vi "Check Condition.vi"(1 "Dictance":dbl, 2 "Condition":dbl, 3 "Reset":bool) -> (0 "Done":bool)   [LabVIEW 2015]
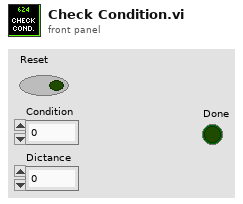
[diagram p1: front panel]
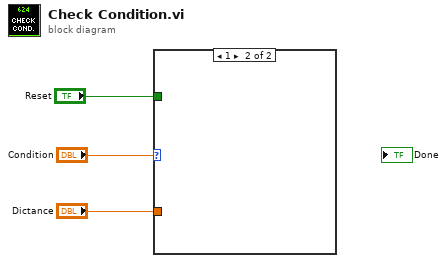
[diagram p0: block diagram]
diagram:
  n1 = case shown="1" "Condition" {
    tunnel: "Dictance" -> [_ _]
    tunnel: "Reset" -> [_ _]
    frame 0, Default {
    }
    frame 1 {
    }
  }
